vi "俄罗斯方块-初始坐标.vi"(11 "输入形状数组":u32[][](array[colorbox])) -> (0 "Y":i8, 1 "X":i8)   [LabVIEW 2016]
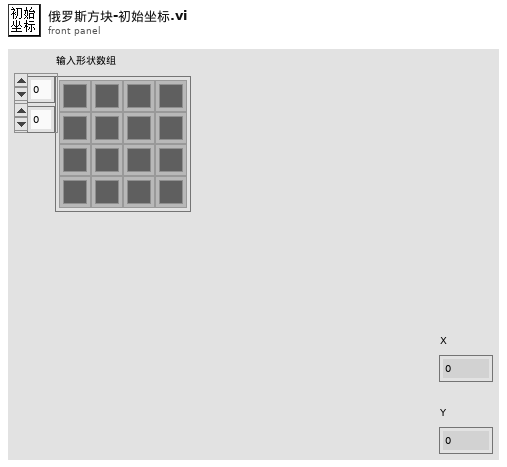
[diagram p1: front panel]
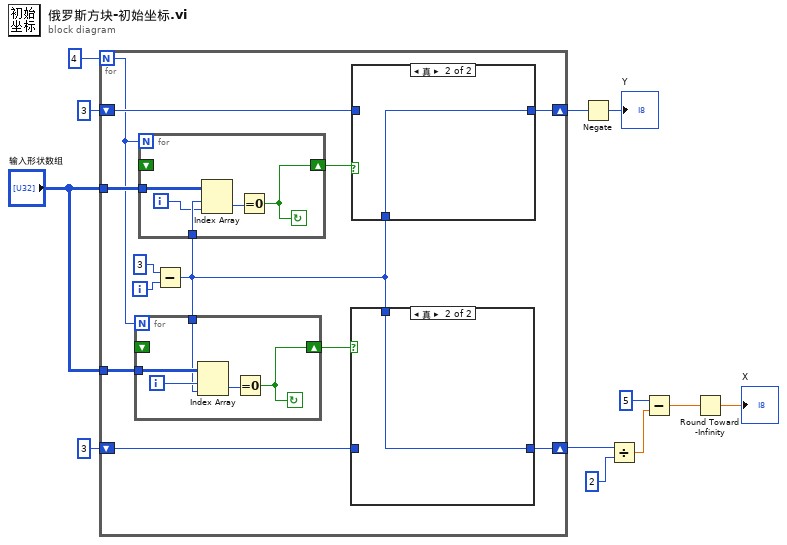
[diagram p0: block diagram]
diagram:
  n1 = for {
    N: 4 -> [w13]
    tunnel: "输入形状数组" -> [w22]
    tunnel: "输入形状数组" -> [w24]
    shift-right: [w18] -> w5
    shift-left: 3 -> [w15]
    shift-right: [w16] -> w8
    shift-left: 3 -> [w14]
    i -> [w21]
    n2 = Subtract(x=3, y=w21) -> (x-y=w17:i32)
    n3 = for {
      N: w13 -> [_]
      tunnel: w24 -> [w38]
      shift-right: [w35] -> w23
      shift-left: _ -> [_]
      tunnel: w17 -> [w34]
      i -> [w37]
      stop <- w35 continue-if-true
      n4 = Index Array(array=w38, index (row)=w37, index (col)=w34) -> (element=w36:u32)
      n5 = Equal To 0?(x=w36) -> (x = 0?=w35:bool)
    }
    n6 = for {
      N: w13 -> [_]
      tunnel: w22 -> [w31]
      shift-right: [w29] -> w19
      shift-left: _ -> [_]
      tunnel: w17 -> [w28]
      i -> [w27]
      stop <- w29 continue-if-true
      n7 = Index Array(array=w31, index (row)=w28, index (col)=w27) -> (element=w30:u32)
      n8 = Equal To 0?(x=w30) -> (x = 0?=w29:bool)
    }
    n9 = case shown="真" w23 {
      tunnel: w17 -> [_ w33]
      tunnel: [w32 w33] -> w18
      tunnel: w15 -> [w32 _]
      frame False {
      }
      frame True {
      }
    }
    n10 = case shown="真" w19 {
      tunnel: w17 -> [_ w26]
      tunnel: [w25 w26] -> w16
      tunnel: w14 -> [w25 _]
      frame False {
      }
      frame True {
      }
    }
  }
  n11 = Negate(x=w8) -> (-x=→"Y":i32)
  n12 = Divide(x=w5, y=i8 2) -> (x/y=w4:dbl)
  n13 = Subtract(x=i8 5, y=w4) -> (x-y=w2:dbl)
  n14 = Round Toward -Infinity(1:w2) -> (0:→"X":dbl)
